vi "Add Step To Front.vi"(6 "Reply Channel":refnum<notifier>, 8 "error in (no error)":errorcluster, 9 "Parameter":variant, 10 "Step Name":string, 11 "Sequencer in":refnum<class "Sequencer.lvclass">) -> (0 "error out":errorcluster)   [LabVIEW 2015, in "Sequencer.lvclass"]
uses:
  Sequencer.lvclass
  Messaging/Message/Message.lvclass
  Single Step Data.ctl
  Sequencer.lvclass/Sequencer.ctl
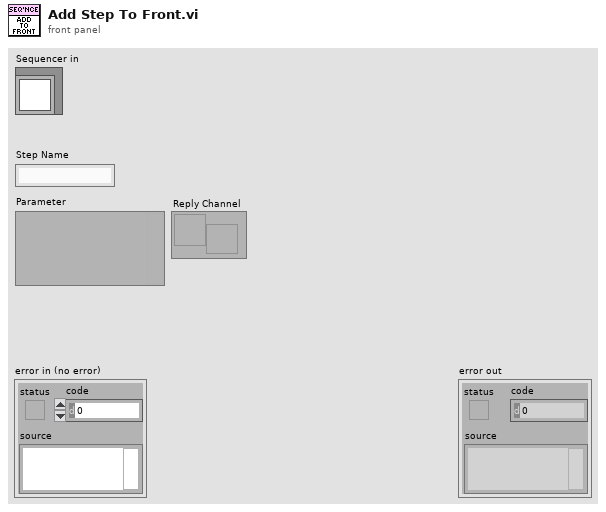
[diagram p1: front panel]
types:
  T1 = typedef "Sequencer.lvclass/Single Step Data.ctl" = cluster{"Step":string, "Parameter":variant, "Reply Channel":refnum<notifier>}
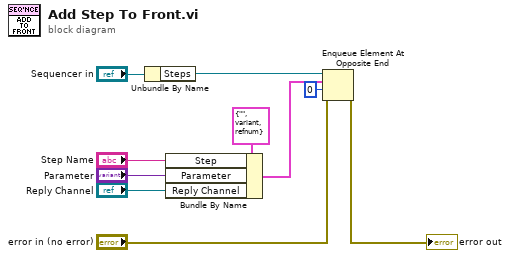
[diagram p0: block diagram]
diagram:
  n1 = Unbundle By Name("Sequencer in") -> ("Steps"=w4:refnum<queue>)
  n2 = Bundle By Name(cluster=T1 {"Step"="", "Parameter"=variant, "Reply Channel"=refnum} ("Cluster"), "Step"="Step Name", "Parameter"="Parameter", "Reply Channel"="Reply Channel") -> (w2:T1)
  n3 = Enqueue Element At Opposite End(queue=w4, element=w2, timeout in ms (-1)=0, error in (no error)="error in (no error)") -> (error out=→"error out":errorcluster)  [unwired: 2 out]
